vi "Calc Init.vi"(8 "error in (no error)":errorcluster, 10 "Config":refnum<class "Channel Config.lvclass">, 11 "Median Calc in":refnum<class "Median Calc.lvclass">) -> (0 "error out":errorcluster, 3 "Median Calc out":refnum<class "Median Calc.lvclass">)   [LabVIEW 2020, in "VolatusCalcs.lvlib" / "Median Calc.lvclass"]
uses:
  Median Calc.lvclass
  Median Calc.lvclass/Median Calc.ctl
  VolatusConfig/VolatusConfigElement/VolatusConfigElement.lvclass
  lv-cdm/CDM-Config/Config Element/Config Element.lvclass
  VolatusConfig/Channel/Channel Config.lvclass
  C:/dev/lv20CE/relink/lv-volatus/VolatusConfig/VolatusConfigElement/VolatusConfigElement.lvclass
  C:/dev/lv20CE/relink/lv-volatus/VolatusConfig/Channel/Channel Config.lvclass
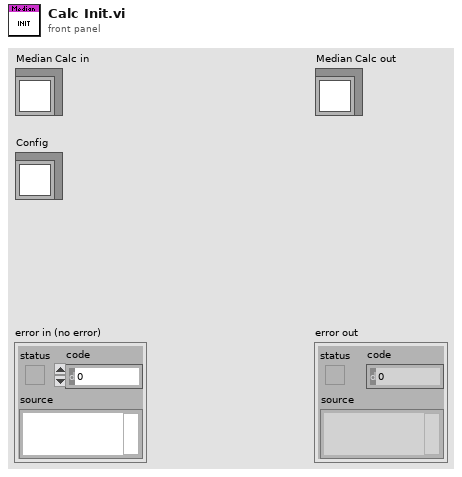
[diagram p1: front panel]
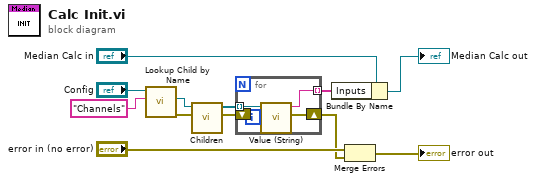
[diagram p0: block diagram]
diagram:
  n1 = call "Lookup Child by Name.vi"("Child Name"="Channels", "VolatusConfigElement in"="Config") -> ("error out"=w8:errorcluster, "Child"=w7:refnum<class "Config Element.lvclass">)  [unwired: 6 in, 2 out]
  n2 = call "Children.vi"("error in (no error)"=w8, "Config Element in"=w7) -> ("error out"=w5:errorcluster, "Elements"=w6:refnum<class "Config Element.lvclass">[])  [unwired: 8 in]
  n3 = for {
    tunnel: w6 -> [w15] mode=indexing
    shift-right: [w14] -> w1
    shift-left: w5 -> [w16]
    tunnel: [w13] -> w3 mode=indexing
    n4 = call "Value (String).vi"("error in (no error)"=w16, "Config Element in"=w15) -> ("error out"=w14:errorcluster, "String Value"=w13:string)  [unwired: 8 in]
  }
  n5 = Bundle By Name(cluster="Median Calc in", "Inputs"=w3) -> (→"Median Calc out":refnum<class "Median Calc.lvclass">)
  n6 = Merge Errors("error in (no error)", w1) -> (→"error out":errorcluster)
